vi "Get Tag Settings from Database.vi"(3 "Tag Settings":T1(array[cluster]) {"Vmax" min=-10.0 max=10.0 step=1.0; "Vmin" min=-10.0 max=10.0 step=1.0}, 8 "Error In":errorcluster, 10 "DeviceName":string, 11 "Database Connection":refnum<k7>) -> (0 "Error Out":errorcluster)   [LabVIEW 2015]
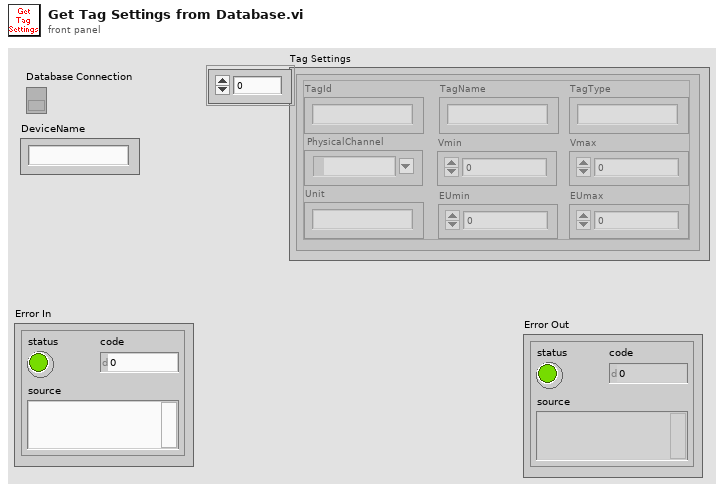
[diagram p1: front panel]
types:
  T1 = cluster{"TagId":string, "TagName":string, "TagType":string, "PhysicalChannel":tag, "Vmin":dbl, "Vmax":dbl, "Unit":string, "EUmin":dbl, "EUmax":dbl}[]
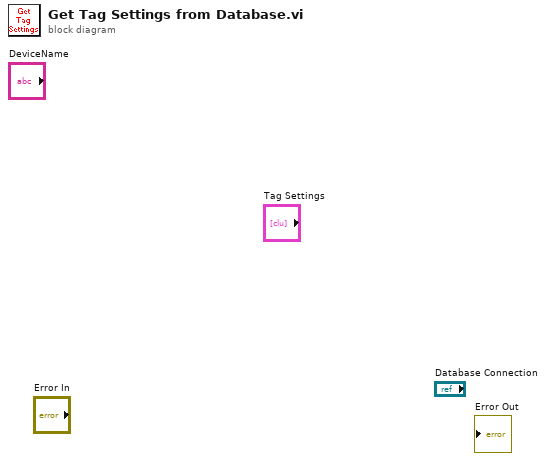
[diagram p0: block diagram]
diagram:
